vi "Write menubar.vi"(8 "error in (no error)":errorcluster, 10 "menubar":refnum<k9>, 11 "Main Class in":refnum<class "Main Class.lvclass">) -> (0 "error out":errorcluster, 3 "Main Class out":refnum<class "Main Class.lvclass">)   [LabVIEW 2019, in "Main Class.lvclass"]
uses:
  Main Class.lvclass
  Main Class.lvclass/Main Class.ctl
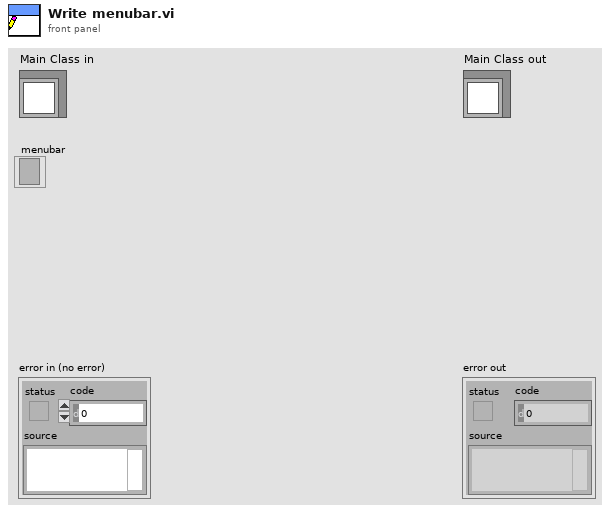
[diagram p1: front panel]
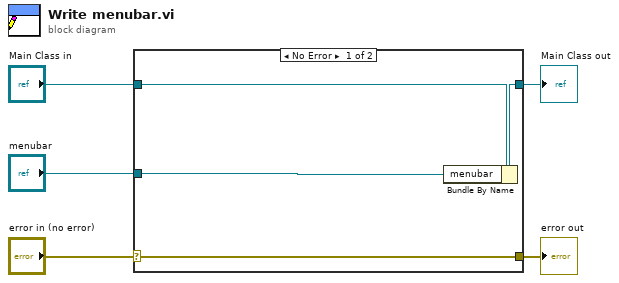
[diagram p0: block diagram]
diagram:
  n1 = case shown="No Error" "error in (no error)" {
    selector: "error in (no error)" -> [w9 w10]
    tunnel: [w9 w10] -> w4
    tunnel: [w7 w11] -> w2
    tunnel: "Main Class in" -> [w8 w11]
    tunnel: "menubar" -> [w6 _]
    frame No Error {
      n2 = Bundle By Name(cluster=w8, "menubar"=w6) -> (w7:refnum<class "Main Class.lvclass">)
    }
    frame Error {
    }
  }
  "error out" <- w4
  "Main Class out" <- w2
